vi "Init Sim.vi"(8 "error in (no error)":errorcluster) -> (0 "error out":errorcluster, 2 "Init":T1, 3 "config path":path)   [LabVIEW 2015]
uses:
  typedefs/init data.ctl
panel:
  in  "Submit spoof":bool
  in  "Submit":bool
  in  "elevator gain":dbl
  in  "aileron gain":dbl
  in  "rudder gain":dbl
  in  "Aircraft Selection":string(combo)="MPX5"
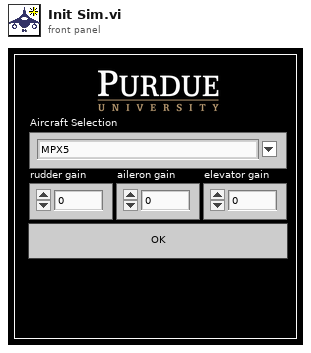
[diagram p1: front panel]
types:
  T1 = typedef "init data.ctl" = cluster{"rudder gain":dbl, "aileron gain":dbl, "elevator gain":dbl, "joystick ID":refnum<k1>}
  T2 = enum32{"Invalid", "Standard", "Closed", "Hidden", "Minimized", "Maximized"}
  T3 = cluster{"axes total":u32, "buttons total":u32, "pov total":u32, "device name":string}
  T4 = cluster{"axes total":u32, "buttons total":u32, "pov total":u32, "device name":string}[]
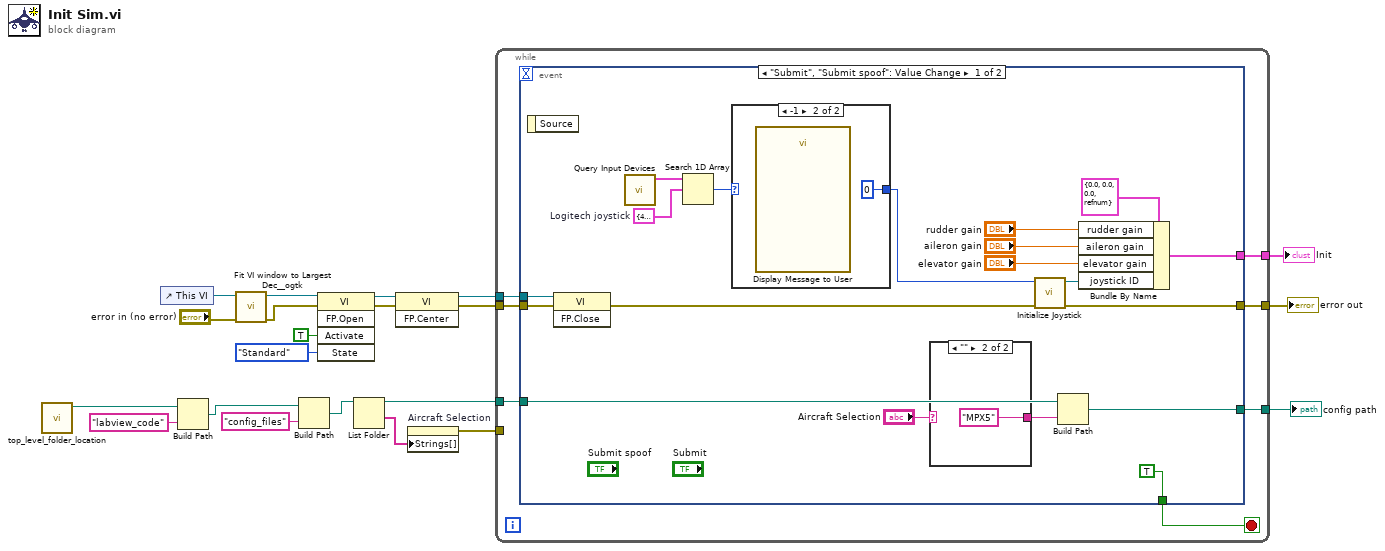
[diagram p0: block diagram]
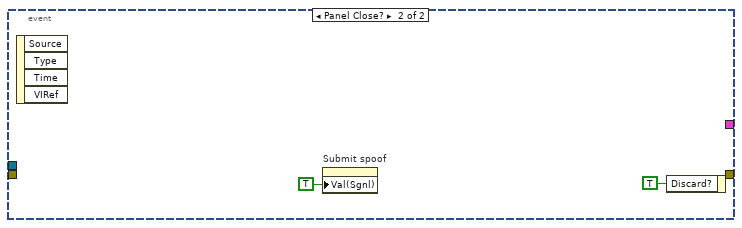
[diagram p4: hidden frame]
diagram:
  n1 = call "top_level_folder_location.vi"() -> ("Parent Folder"=w19:path)  [unwired: 11 in]
  n2 = control-ref of="This VI"() -> (w8:refnum<vi>)
  n3 = Build Path(base path=w19, name or relative path="labview_code") -> (appended path=w17:path)
  n4 = call "Fit VI window to Largest Dec__ogtk.vi"("error in (no error)"="error in (no error)", "VI Ref (calling VI)"=w8) -> ("error out"=w6:errorcluster, "dup VI Ref"=w7:refnum<vi>)  [unwired: 4 in]
  n5 = Build Path(base path=w17, name or relative path="config_files") -> (appended path=w20:path)
  n6 = invoke class="VI" method="FP.Open"(reference=w7, error in=w6, "Activate"=TRUE ("Activate?"), "State"=T2."Standard") -> (reference out=w10:refnum<vi>, error out=w5:errorcluster)  [unwired: 1 in, 3 out]
  n7 = List Folder(path=w20) -> (path out=w15:path, folder names=w1:string[])  [unwired: 3 in, 2 out]
  n8 = invoke class="VI" method="FP.Center"(reference=w10, error in=w5) -> (reference out=w4:refnum<vi>, error out=w9:errorcluster)  [unwired: 1 in, 1 out]
  n9 = property on="Aircraft Selection" class="CmbBox"("Strings[]"=w1) -> (error out=w16:errorcluster)  [unwired: 2 in, 1 out]
  n10 = while {
    tunnel: w16 -> [_]
    tunnel: w15 -> [w27]
    tunnel: [w26] -> w14
    tunnel: [w25] -> w13
    tunnel: w9 -> [w22]
    tunnel: [w24] -> w3
    tunnel: w4 -> [w23]
    stop <- w28 stop-if-true
    n11 = event shown="[0] \"Submit\", \"Submit spoof\": Value Change" {
      selector: _ -> [_ _]
      dyn-events: _ -> [_ _]
      timeout: _ -> [_ _]
      tunnel: [TRUE _] -> w28
      tunnel: w27 -> [w42 _]
      tunnel: [w41 _] -> w26
      tunnel: [w40 _] -> w25
      tunnel: [w38 _] -> w24
      tunnel: w23 -> [w37 _]
      tunnel: w22 -> [w36 _]
      event "Submit", "Submit spoof": Value Change {
        w31 = T3 {"axes total"=4, "buttons total"=12, "pov total"=1, "device name"="Logitech Extreme 3D"}  # Logitech joystick
        n12 = event-data() -> ()  [unwired: 1 in, 1 out]
        n13 = invoke class="VI" method="FP.Close"(reference=w37, error in=w36) -> (error out=w35:errorcluster)  [unwired: 1 in, 2 out]
        n14 = call <vilib>:"Query Input Devices.vi"() -> ("joystick info"=w30:T4)  [unwired: 8 in, 3 out]
        n15 = Search 1D Array(1D array=w30, element=w31) -> (index of element=w32:i32)  [unwired: 1 in]
        n16 = case shown="-1" w32 {
          selector: w32 -> [w48 _]
          tunnel: [w48 0 ("index of element")] -> w29
          frame Default {
          }
          frame -1 {
            n17 = call "Display Message to User"() -> ()  [unwired: 10 in, 2 out]
          }
        }
        n18 = case shown="\"\"" "Aircraft Selection" {
          selector: "Aircraft Selection" -> [w50 _]
          tunnel: [w50 "MPX5"] -> w33
          frame Default {
          }
          frame "" {
          }
        }
        n19 = call <vilib>:"Initialize Joystick.vi"("error in (no error)"=w35, "device index"=w29) -> ("error out"=w38:errorcluster, "device ID"=w47:refnum<k1>)  [unwired: 8 in]
        n20 = Build Path(base path=w42, name or relative path=w33) -> (appended path=w41:path)
        n21 = Bundle By Name(cluster=T1 {"rudder gain"=0.0, "aileron gain"=0.0, "elevator gain"=0.0, "joystick ID"=refnum}, "rudder gain"="rudder gain", "aileron gain"="aileron gain", "elevator gain"="elevator gain", "joystick ID"=w47) -> (w40:T1)
      }
      event Panel Close? {
        n22 = event-data() -> ()  [unwired: 1 in, 4 out]
        n23 = property on="Submit spoof" class="Bool (strict)"("Val(Sgnl)"=TRUE ("Value (Signaling)")) -> ()  [unwired: 2 in, 2 out]
        n24 = event-data("Discard?"=TRUE) -> ()  [unwired: 1 in, 1 out]
      }
    }
  }
  "config path" <- w14
  "Init" <- w13
  "error out" <- w3
